vi "test_libssh2_channel_exec.vi"() -> ()   [LabVIEW 2017, in "integration_tests.lvlib"]
uses:
  integration_tests.lvlib
  libssh2/libssh2_channel_open_ex.vi
  libssh2/libssh2_channel_process_startup.vi
  support/support.lvlib
  libssh2/libssh2.lvlib
  <vilib>/PNR/Transparent Assertions/Transparent Assertions/Transparent Assertions.lvlib
panel:
  out "error out":errorcluster
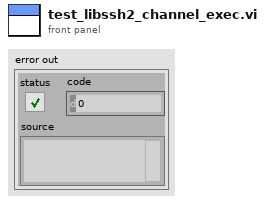
[diagram p1: front panel]
types:
  T1 = typedef "libssh2.lvlib/Session Refnum.ctl" = refnum<k1>
  T2 = typedef "libssh2.lvlib/Channel Refnum.ctl" = refnum<k1>
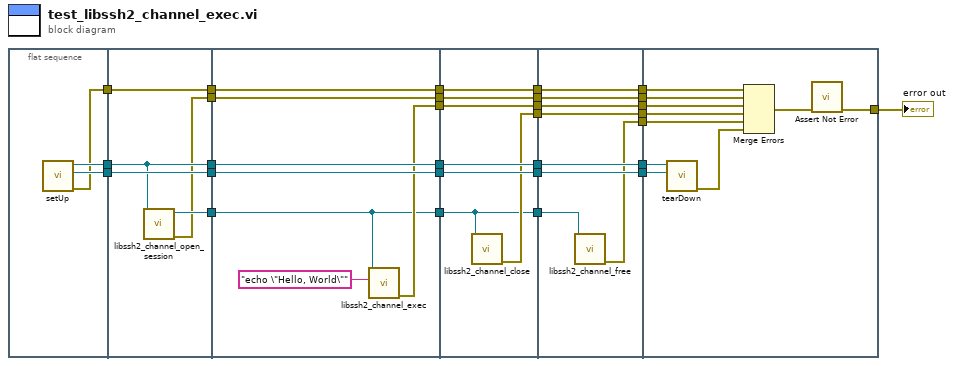
[diagram p0: block diagram]
diagram:
  n1 = flat-sequence {
    tunnel: [w32] -> w29
    tunnel: [w31] -> w28
    tunnel: [w30] -> w27
    tunnel: w29 -> [w36]
    tunnel: w28 -> [w37]
    tunnel: [w36] -> w26
    tunnel: [w37] -> w25
    tunnel: [w35] -> w24
    tunnel: w27 -> [w34]
    tunnel: [w34] -> w23
    tunnel: [w33] -> w22
    tunnel: w26 -> [w44]
    tunnel: [w44] -> w7
    tunnel: w25 -> [w43]
    tunnel: [w43] -> w6
    tunnel: w24 -> [w38]
    tunnel: w23 -> [w42]
    tunnel: [w42] -> w5
    tunnel: w22 -> [w40]
    tunnel: [w40] -> w4
    tunnel: [w39] -> w3
    tunnel: [w38] -> w2
    tunnel: w7 -> [w51]
    tunnel: w6 -> [w50]
    tunnel: [w51] -> w21
    tunnel: [w50] -> w20
    tunnel: [w49] -> w19
    tunnel: w5 -> [w48]
    tunnel: [w48] -> w18
    tunnel: w4 -> [w47]
    tunnel: [w47] -> w17
    tunnel: w3 -> [w46]
    tunnel: [w46] -> w16
    tunnel: w2 -> [w45]
    tunnel: [w45] -> w1
    tunnel: w21 -> [w59]
    tunnel: w20 -> [w58]
    tunnel: [w59] -> w15
    tunnel: [w58] -> w14
    tunnel: [w57] -> w13
    tunnel: w19 -> [w56]
    tunnel: [w56] -> w12
    tunnel: w18 -> [w55]
    tunnel: [w55] -> w11
    tunnel: w17 -> [w54]
    tunnel: [w54] -> w10
    tunnel: w16 -> [w53]
    tunnel: [w53] -> w9
    tunnel: w1 -> [w52]
    tunnel: w15 -> [w69]
    tunnel: w14 -> [w68]
    tunnel: [w67] -> w8
    tunnel: w13 -> [w65]
    tunnel: w12 -> [w64]
    tunnel: w11 -> [w63]
    tunnel: w10 -> [w61]
    tunnel: w9 -> [w60]
    frame #0 {
      n2 = call "setUp.vi"() -> ("error out"=w30:errorcluster, "connection ID"=w31:refnum<k5>, "session"=w32:T1)  [unwired: 9 in]
    }
    frame #1 {
      n3 = call "libssh2_channel_open_session.vi"("session"=w36) -> ("error out"=w33:errorcluster, "channel"=w35:T2)  [unwired: 9 in]
    }
    frame #2 {
      n4 = call "libssh2_channel_exec.vi"("command"="echo \"Hello, World\"", "channel"=w38) -> ("error out"=w39:errorcluster)  [unwired: 9 in]
    }
    frame #3 {
      n5 = call "libssh2_channel_close.vi"("channel"=w45) -> ("error out"=w49:errorcluster)  [unwired: 10 in]
    }
    frame #4 {
      n6 = call "libssh2_channel_free.vi"("channel"=w52) -> ("error out"=w57:errorcluster)  [unwired: 10 in]
    }
    frame #5 {
      n7 = call "tearDown.vi"("connection ID"=w68, "session"=w69) -> ("error out"=w66:errorcluster)  [unwired: 9 in]
      n8 = Merge Errors(w63, w61, w60, w64, w65, w66) -> (w62:errorcluster)
      n9 = call <vilib>:"Assert Not Error.vi"("error in (no error)"=w62) -> ("error out"=w67:errorcluster)  [unwired: 10 in]
    }
  }
  "error out" <- w8
